vi "GetVelocitySetpoint.vi"(11 "DriveBase.lvclass":refnum<class "DriveBase.lvclass">) -> (1 "leftVelocitySetpointOutput":dbl, 2 "rightVelocitySetpointOutput":dbl, 3 "DriveBase.lvclass 2":refnum<class "DriveBase.lvclass">)   [LabVIEW 2016, in "DriveBase.lvclass"]
uses:
  DriveBase.lvclass
  DriveBase.lvclass/DriveBase.ctl
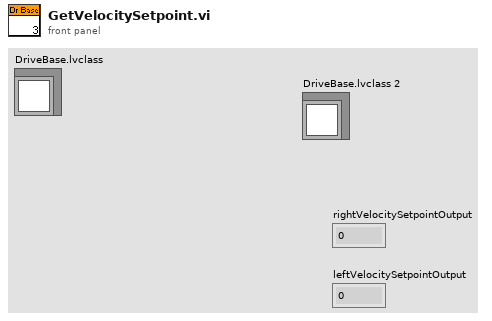
[diagram p1: front panel]
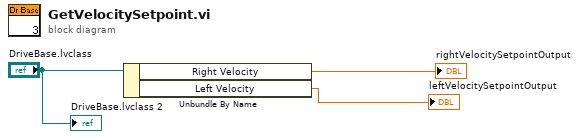
[diagram p0: block diagram]
diagram:
  n1 = Unbundle By Name("DriveBase.lvclass") -> ("Right Velocity"=→"rightVelocitySetpointOutput":dbl, "Left Velocity"=→"leftVelocitySetpointOutput":dbl)
  "DriveBase.lvclass 2" <- "DriveBase.lvclass"
